vi "Configure Noise Level.vi"(8 "error in":errorcluster, 10 "level":dbl, 11 "fpga session in":refnum<k20>) -> (0 "error out":errorcluster, 3 "fpga session out":refnum<k20>)   [LabVIEW 2017, in "Lock-In Amplifier Example Host.lvlib"]
uses:
  Lock-In Amplifier Example Host.lvlib
  fpga type.ctl
  <vilib>/Utility/error.llb/Error Cluster From Error Code.vi
  <vilib>/rvi/errors/niLvFpgaAdjustHostInterfaceError.vi
  <vilib>/rvi/interface/nirviReadWriteControl/nirviReadWriteControl.xnode
  NiFpgaLv.dll
  <vilib>/rvi/interface/Simulation/niFpgaSimulationCallBeginRW.vi
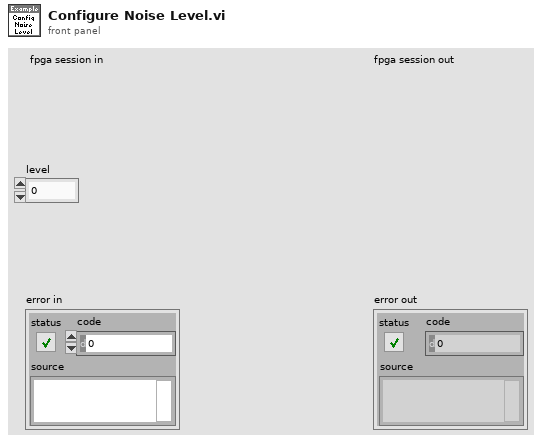
[diagram p1: front panel]
types:
  T1 = typedef "Lock-In Amplifier Example Host.lvlib/fpga type.ctl" = refnum<k20>
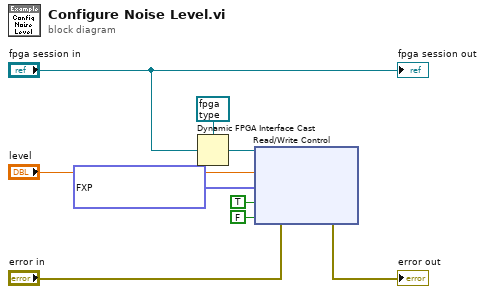
[diagram p0: block diagram]
diagram:
  n1 = Dynamic FPGA Interface Cast(Session In=T1 refnum ("fpga type"), Type="fpga session in") -> (Session Out=w7:T1)
  n2 = xnode "Read/Write Control"("FPGA VI Reference In"=w7, "error in"="error in", "ao.noise gain 3"="level", "ao.noise seeds 3"=fxp<+,23,23>[] [24324.0, 43244.0], "ao.reset 3"=TRUE, "ao.reset 3"=FALSE) -> ("error out"=→"error out":errorcluster)  [unwired: 1 out]
  "fpga session out" <- "fpga session in"
